vi "DeactivateAnalogPositionSettingValue.vi"(4 "error in (no error)":errorcluster, 6 "analogInputNumber":u16, 7 "axis in":cluster{"keyHandle":u32, "nodeId":u16}={"keyHandle"=0, "nodeId"=1}) -> (0 "error out":errorcluster, 3 "axis out":cluster{"keyHandle":u32, "nodeId":u16}={"keyHandle"=0, "nodeId"=1})   [LabVIEW 2017, in "maxonEPOS.lvlib"]
doc: "<B>DeactivateAnalogPositionSettingValue</B> disables the selected analog input for analog position setpoint."
uses:
  Examples/maxonEPOS.lvlib
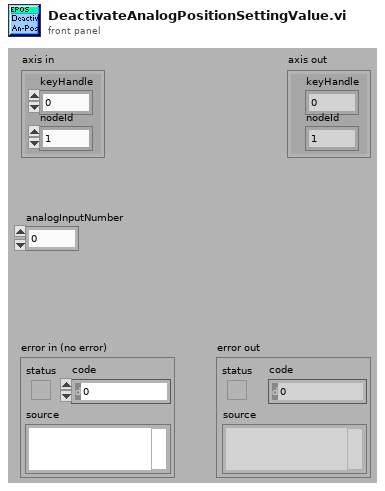
[diagram p1: front panel]
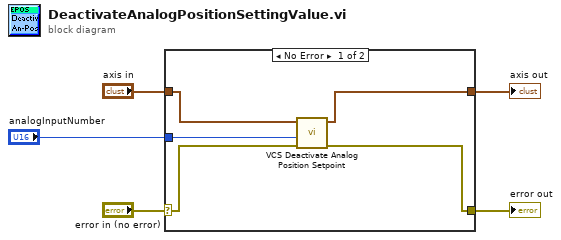
[diagram p0: block diagram]
diagram:
  n1 = case shown="No Error" "error in (no error)" {
    selector: "error in (no error)" -> [w10 w12]
    tunnel: [w6 w12] -> w4
    tunnel: [w7 w11] -> w3
    tunnel: "axis in" -> [w9 w11]
    tunnel: "analogInputNumber" -> [w8 _]
    frame No Error {
      n2 = call "VCS Deactivate Analog Position Setpoint.vi"("error in (no error)"=w10, "analogInputNumber"=w8, "axis in"=w9) -> ("error out"=w6:errorcluster, "axis out"=w7:cluster{"keyHandle":u32, "nodeId":u16})  [unwired: 7 in]
    }
    frame Error {
    }
  }
  "error out" <- w4
  "axis out" <- w3
